vi "Basic double map example.vi"() -> ()   [LabVIEW 2021]
uses:
  CIFChannels/CIFChannels.lvclass
  Channels/Test Channel/Test Channel.lvclass
  D:/dev/CIF-LVCore/src/CIFUtilities/CIFChannels/CIFChannels.lvclass
  typedef/String to U16 Map.ctl
  typedef/U16 to Channel Map.ctl
  Channels/Test Channel/Test Channel.lvclass/Test Channel.ctl
  CIFChannels/CIFChannels.lvclass/CIFChannels.ctl
  D:/dev/CIF-LVCore/src/Channels/Test Channel/Test Channel.lvclass
  CIFChannelMng.lvclass
panel:
  out "error out":errorcluster
  out "Name":string
  out "test":dbl
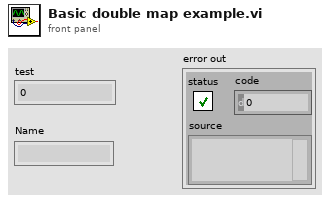
[diagram p1: front panel]
types:
  T1 = typedef "CIFChannelMng.lvclass/U16 to Channel Map.ctl" = map{u16, refnum<class "CIFChannels.lvclass">}
  T2 = typedef "CIFChannelMng.lvclass/String to U16 Map.ctl" = map{string, u16}
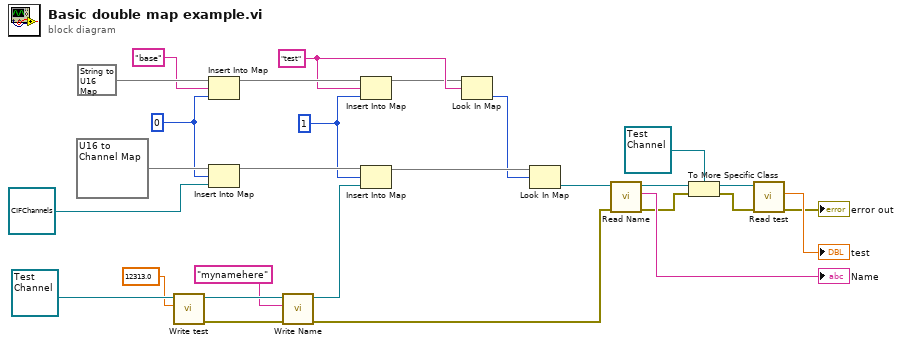
[diagram p0: block diagram]
diagram:
  w15 = u16 1 ("value")
  w18 = u16 0 ("value")
  w23 = "test" ("key")
  n1 = call "Write test.vi"("test"=12313.0, "Test Channel in"=refnum<class "Test Channel.lvclass"> refnum ("Test Channel.lvclass")) -> ("error out"=w5:errorcluster, "Test Channel out"=w11:refnum<class "Test Channel.lvclass">)  [unwired: 8 in]
  n2 = Insert Into Map(map in=T2 {} ("String Key Map"), key="base", value=w18) -> (map out=w26:T2)  [unwired: 2 out]
  n3 = Insert Into Map(map in=T1 {} ("U16 to Class Map"), key=w18, value=refnum<class "CIFChannels.lvclass"> refnum ("CIFChannels.lvclass")) -> (map out=w16:T1)  [unwired: 2 out]
  n4 = call "Write Name.vi"("error in (no error)"=w5, "Name"="mynamehere", "CIFChannels in"=w11) -> ("error out"=w4:errorcluster, "CIFChannels out"=w10:refnum<class "Test Channel.lvclass">)  [unwired: 7 in]
  n5 = Insert Into Map(map in=w26, key=w23, value=w15) -> (map out=w14:T2)  [unwired: 2 out]
  n6 = Insert Into Map(map in=w16, key=w15, value=w10) -> (map out=w13:T1)  [unwired: 2 out]
  n7 = Look In Map(map=w14, key=w23) -> (value=w12:u16)  [unwired: 1 in, 1 out]
  n8 = Look In Map(map=w13, key=w12) -> (value=w8:refnum<class "CIFChannels.lvclass">)  [unwired: 1 in, 1 out]
  n9 = call "Read Name.vi"("error in (no error)"=w4, "CIFChannels in"=w8) -> ("error out"=w3:errorcluster, "Name"=→"Name":string, "CIFChannels out"=w6:refnum<class "CIFChannels.lvclass">)  [unwired: 7 in]
  n10 = To More Specific Class(target class=refnum<class "Test Channel.lvclass"> refnum ("Test Channel.lvclass"), reference=w6, error in=w3) -> (specific class reference=w22:refnum<class "Test Channel.lvclass">, error out=w2:errorcluster)
  n11 = call "Read test.vi"("error in (no error)"=w2, "Test Channel in"=w22) -> ("error out"=→"error out":errorcluster, "test"=→"test":dbl)  [unwired: 7 in, 1 out]
